vi "Process Banana Message.vi"(8 "error in (no error)":errorcluster, 10 "Message":T3, 11 "Tamer in":refnum<class "Tamer.lvclass">) -> (0 "error out":errorcluster, 1 "Propagate Banana?":bool, 2 "Internal Banana":T1, 3 "Tamer out":refnum<class "Tamer.lvclass">)   [LabVIEW 2020, in "Tamer.lvlib" / "Tamer.lvclass"]
uses:
  Tamer.lvclass
  Run Utilities/TypeDefs/Messages/Banana Message.ctl
  Run Utilities/TypeDefs/Return Code.ctl
  Internatl Banana.ctl
  Tamer.lvclass/Tamer.ctl
  TALOS/TALOS_PPL.lvlibp/Guardian/Guardian/Requests.ctl
  Run Utilities/Run Utilities.lvlib
  TALOS/TALOS_PPL.lvlibp
  TALOS/TALOS_PPL.lvlibp/Guardian/Guardian/Guardian.lvclass
  TALOS/TALOS_PPL.lvlibp/Father of all uServices/Father of all uServices/Father of all uServices.lvclass
  C:/Users/aegis/Documents/CIRCUS/TALOS/TALOS_PPL.lvlibp/Father of all uServices/Father of all uServices/Father of all uServices.lvclass
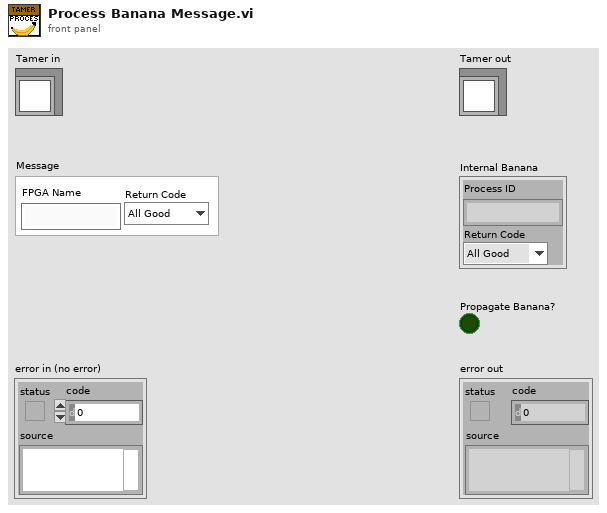
[diagram p1: front panel]
types:
  T1 = typedef "Tamer.lvlib/Tamer.lvclass/Internatl Banana.ctl" = cluster{"Process ID":string, "Return Code":T2}
  T2 = typedef "Run Utilities.lvlib/Return Code.ctl" = enum16{"All Good", "Retry", "Skip", "Skip All", "ABORT"}
  T3 = typedef "Run Utilities.lvlib/Banana Message.ctl" = cluster{"FPGA Name":string, "Return Code":T2}
  T4 = typedef "TALOS_PPL.lvlibp/Guardian.lvlib/Guardian.lvclass/Requests.ctl" = enum16{"Ready to Launch", "Start RUN", "Stop RUN", "Update DAQ Params", "Update Error Listbox", "Update Run Status", "Update Kasli Log", "Run Stopped with Errors", "Switch uS View"}
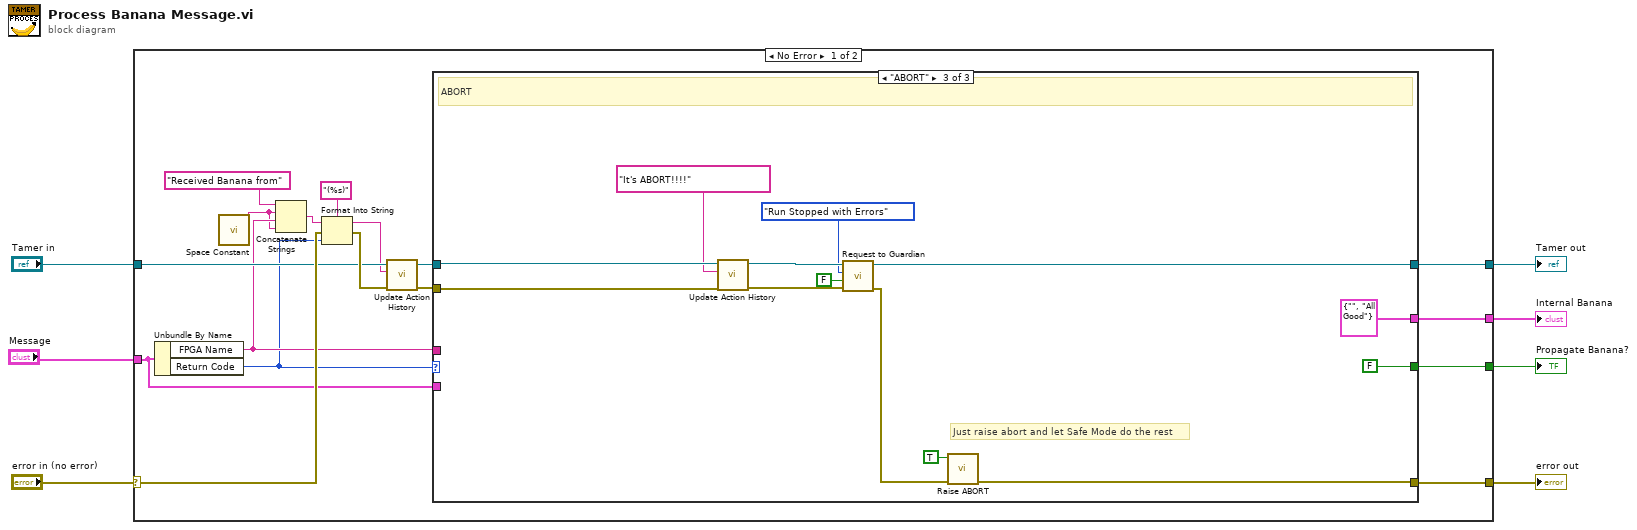
[diagram p0: block diagram]
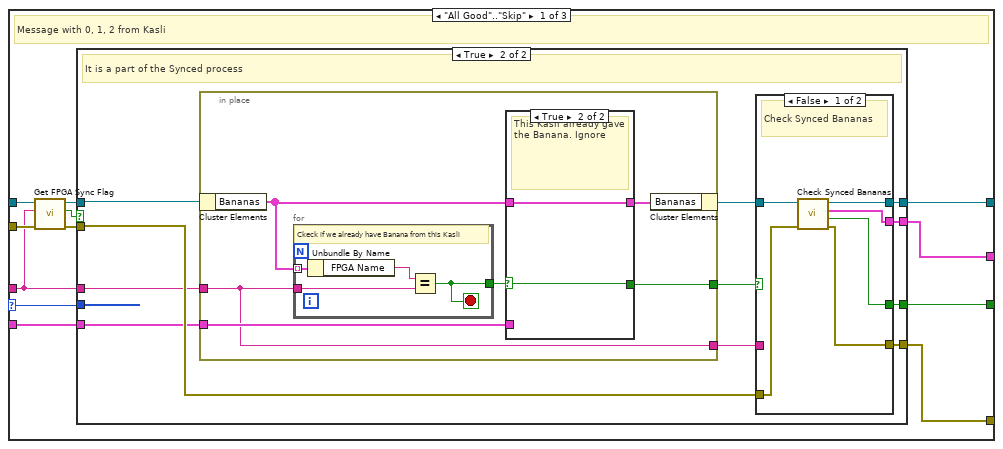
[diagram p2: hidden frame]
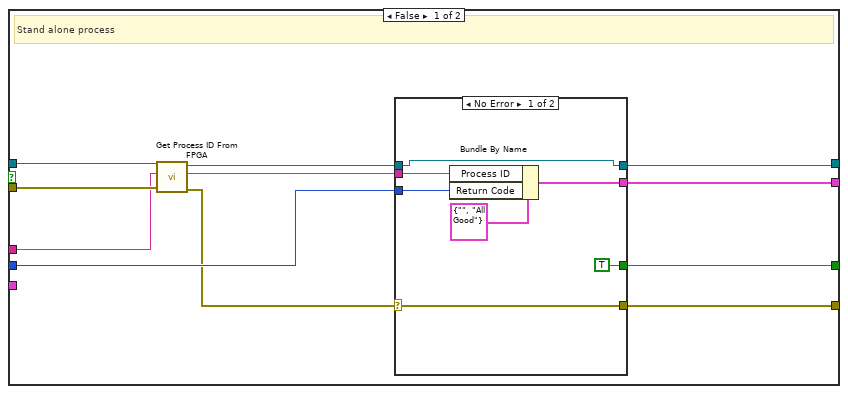
[diagram p3: hidden frame]
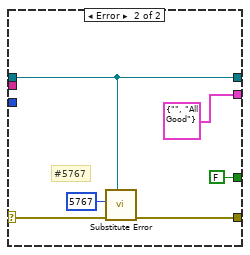
[diagram p4: hidden frame]
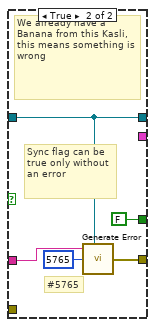
[diagram p5: hidden frame]
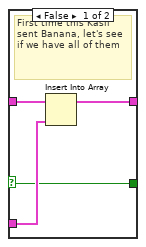
[diagram p6: hidden frame]
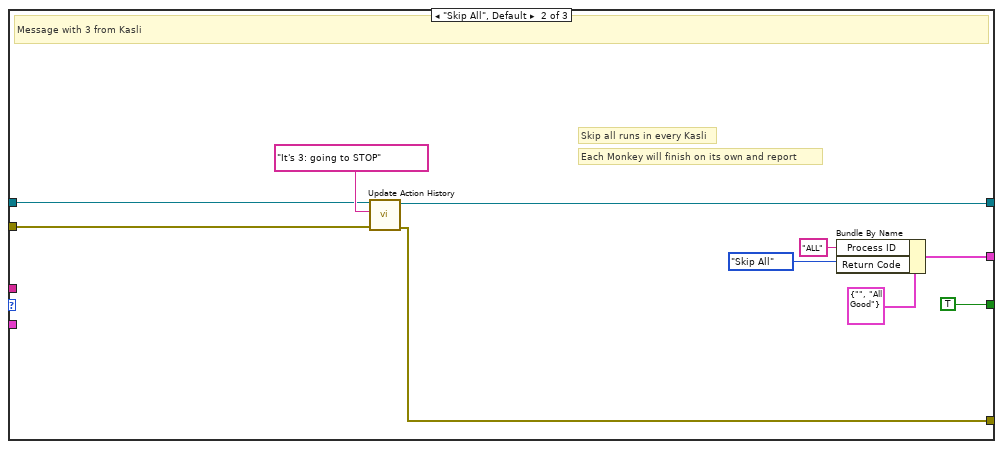
[diagram p7: hidden frame]
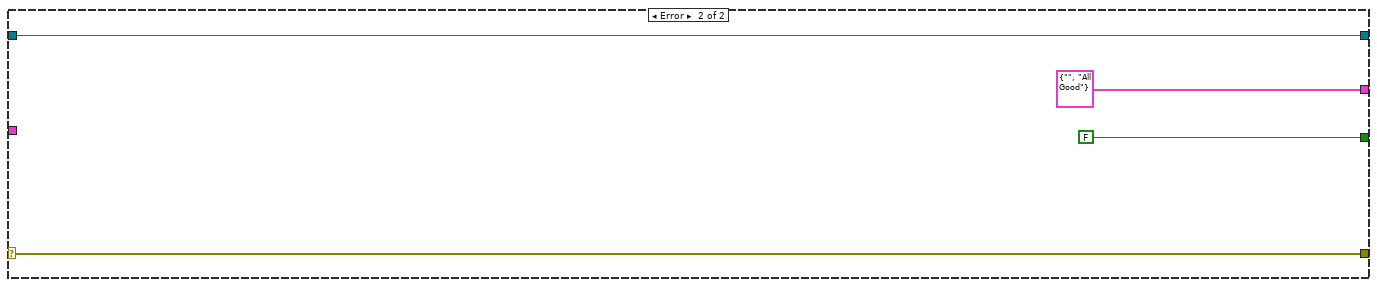
[diagram p8: hidden frame]
diagram:
  n1 = case shown="No Error" "error in (no error)" {
    selector: "error in (no error)" -> [w23 w125]
    tunnel: [w15 w125] -> w6
    tunnel: [w21 w124] -> w4
    tunnel: "Tamer in" -> [w17 w124]
    tunnel: "Message" -> [w22 _]
    tunnel: [w20 T1 {"Process ID"="", "Return Code"=enum."All Good"} ("Internal Banana")] -> w1
    tunnel: [w19 FALSE ("Propagate Banana?")] -> w2
    frame No Error {
      n2 = Unbundle By Name(w22) -> ("FPGA Name"=w16:string, "Return Code"=w13:T2)
      n3 = call <vilib>:"Space Constant.vi"() -> ("String"=w10:string)
      n4 = Concatenate Strings("Received Banana from" ("string"), w10, w16, w10) -> (w14:string)
      n5 = Format Into String(format string="(%s)", initial string=w14, error in=w23, w13) -> (resulting string=w12:string, error out=w24:errorcluster)
      n6 = call-dynamic "Update Action History.vi"("error in (no error)"=w24, "Action"=w12, "Tamer in"=w17) -> ("error out"=w8:errorcluster, "Tamer out"=w9:refnum<class "Tamer.lvclass">)  [unwired: 7 in]
      n7 = case shown="\"ABORT\"" w13 {
        selector: w13 -> [w31 _ _]
        tunnel: w9 -> [w29 w102 w116]
        tunnel: w8 -> [w28 w100 w117]
        tunnel: w22 -> [w36 _ _]
        tunnel: w16 -> [w25 _ _]
        tunnel: [w35 w101 w112] -> w21
        tunnel: [w34 w99 w121] -> w15
        tunnel: [w33 w105 T1 {"Process ID"="", "Return Code"=enum."All Good"} ("Internal Banana")] -> w20
        tunnel: [w32 TRUE ("Propagate Banana?") FALSE ("Propagate Banana?")] -> w19
        frame "All Good".."Skip" {
          # "Message with 0, 1, 2 from Kasli"
          n8 = call-dynamic "Get FPGA Sync Flag.vi"("error in (no error)"=w28, "FPGA Name"=w25, "Tamer in"=w29) -> ("error out"=w27:errorcluster, "FPGA Sync Flag"=w26:bool, "Tamer out"=w30:refnum<class "Tamer.lvclass">)  [unwired: 6 in]
          n9 = case shown="True" w26 {
            tunnel: [w39 w66] -> w35
            tunnel: [w38 w68] -> w34
            tunnel: w25 -> [w45 w62]
            tunnel: w30 -> [w47 w61]
            tunnel: w27 -> [w46 w71]
            tunnel: w36 -> [_ w70]
            tunnel: w31 -> [w43 _]
            tunnel: [w42 w64] -> w33
            tunnel: [w37 w63] -> w32
            frame False {
              # "Stand alone process"
              n10 = call-dynamic "Get Process ID From FPGA.vi"("error in (no error)"=w46, "FPGA Name"=w45, "Tamer in"=w47) -> ("error out"=w41:errorcluster, "Process ID"=w44:string, "Tamer out"=w40:refnum<class "Tamer.lvclass">)  [unwired: 6 in]
              n11 = case shown="No Error" w41 {
                selector: w41 -> [w49 w60]
                tunnel: w44 -> [w50 _]
                tunnel: w43 -> [w53 _]
                tunnel: [w52 T1 {"Process ID"="", "Return Code"=enum."All Good"} ("Internal Banana")] -> w42
                tunnel: w40 -> [w48 w58]
                tunnel: [w48 w58] -> w39
                tunnel: [w49 w59] -> w38
                tunnel: [TRUE ("Propagate Banana?") FALSE ("Propagate Banana?")] -> w37
                frame No Error {
                  n12 = Bundle By Name(cluster=T1 {"Process ID"="", "Return Code"=enum."All Good"} ("Internal Banana"), "Process ID"=w50, "Return Code"=w53) -> (w52:T1)
                }
                frame Error {
                  # "#5767"
                  n13 = call "Substitute Error.vi"("LabVIEW Object"=w58, "error in (no error)"=w60, "Error Code"=5767) -> ("error out"=w59:errorcluster)  [unwired: 8 in]
                }
              }
            }
            frame True {
              # "It is a part of the Synced process"
              n14 = in-place {
                in-place-border: w62 -> [w83]
                in-place-border: w70 -> [w85]
                in-place-border: [w84] -> w69
                in-place-border: [w83] -> w65
                n15 = in-place-cluster #1(w61) -> ("Bananas"=w87:T3[])
                n16 = for {
                  tunnel: w87 -> [w98] mode=indexing
                  tunnel: [w96] -> w88
                  tunnel: w83 -> [w95]
                  stop <- w96 stop-if-true
                  # "Ckeck if we already have Banana from this Kasli"
                  n17 = Unbundle By Name(w98) -> ("FPGA Name"=w97:string)
                  n18 = Equal?(x=w97, y=w95) -> (x = y?=w96:bool)
                }
                n19 = case shown="True" w88 {
                  selector: w88 -> [w89 w93]
                  tunnel: w87 -> [w92 w94]
                  tunnel: [w90 w94] -> w86
                  tunnel: w85 -> [w91 _]
                  tunnel: [w89 w93] -> w84
                  frame False {
                    # "First time this Kasli sent Banana, let's see if we have all of them"
                    n20 = Insert Into Array(array=w92, new element=w91) -> (w90:T3[])  [unwired: 1 in]
                  }
                  frame True {
                    # "This Kasli already gave the Banana. Ignore"
                  }
                }
                n21 = in-place-cluster #1("Bananas"=w86) -> (w67:refnum<class "Tamer.lvclass">)
              }
              n22 = case shown="False" w69 {
                tunnel: [w75 w81] -> w68
                tunnel: w67 -> [w77 w80]
                tunnel: [w74 w80] -> w66
                tunnel: w65 -> [_ w79]
                tunnel: w71 -> [w76 _]
                tunnel: [w73 _] -> w64
                tunnel: [w72 FALSE ("Propagate Banana?")] -> w63
                frame False {
                  # "Check Synced Bananas"
                  n23 = call-dynamic "Check Synced Bananas.vi"("error in (no error)"=w76, "Tamer in"=w77) -> ("error out"=w75:errorcluster, "Propagate Banana?"=w72:bool, "Internal Banana"=w73:T1, "Tamer out"=w74:refnum<class "Tamer.lvclass">)  [unwired: 6 in]
                }
                frame True {
                  # "Sync flag can be true only without an error"
                  # "#5765"
                  # "We already have a Banana from this Kasli, this means something is wrong"
                  n24 = call "Generate Error.vi"("Optional String"=w79, "Class"=w80, "Error Code"=5765) -> ("error out"=w81:errorcluster)  [unwired: 4 in]
                }
              }
            }
          }
        }
        frame "Skip All", Default {
          # "Each Monkey will finish on its own and report"
          # "Skip all runs in every Kasli"
          # "Message with 3 from Kasli"
          n25 = call-dynamic "Update Action History.vi"("error in (no error)"=w100, "Action"="It's 3: going to STOP", "Tamer in"=w102) -> ("error out"=w99:errorcluster, "Tamer out"=w101:refnum<class "Tamer.lvclass">)  [unwired: 7 in]
          n26 = Bundle By Name(cluster=T1 {"Process ID"="", "Return Code"=enum."All Good"} ("Internal Banana"), "Process ID"="ALL", "Return Code"=Return_Code."Skip All") -> (w105:T1)
        }
        frame "ABORT" {
          # "Just raise abort and let Safe Mode do the rest"
          # "ABORT"
          n27 = call-dynamic "Update Action History.vi"("error in (no error)"=w117, "Action"="It's ABORT!!!!", "Tamer in"=w116) -> ("error out"=w110:errorcluster, "Tamer out"=w113:refnum<class "Tamer.lvclass">)  [unwired: 7 in]
          n28 = call "Request to Guardian.vi"("error in (no error)"=w110, "Data"=FALSE, "Requests"=Requests."Run Stopped with Errors", "Father of all uServices in"=w113) -> ("error out"=w109:errorcluster, "Father of all uServices out"=w112:refnum<class "Tamer.lvclass">)  [unwired: 6 in]
          n29 = call "Raise ABORT.vi"("error in"=w109, "ABORT?"=TRUE) -> ("error out"=w121:errorcluster)  [unwired: 9 in]
        }
      }
    }
    frame Error {
    }
  }
  "error out" <- w6
  "Tamer out" <- w4
  "Propagate Banana?" <- w2
  "Internal Banana" <- w1
